vi "Image_Processing_Edge_Detection.vi"() -> ()   [LabVIEW 2015]
uses:
  <vilib>/picture/picture.llb/imagedata.ctl
  <vilib>/Analysis/2dsp.llb/2D Convolution (DBL).vi
  <vilib>/picture/picture.llb/Draw 8-Bit Pixmap.vi
  <vilib>/Analysis/NI_AALPro.lvlib
panel:
  out "new picture 2":picture
  out "new picture":picture
  out "image data":T1
  in  "Input Image":path
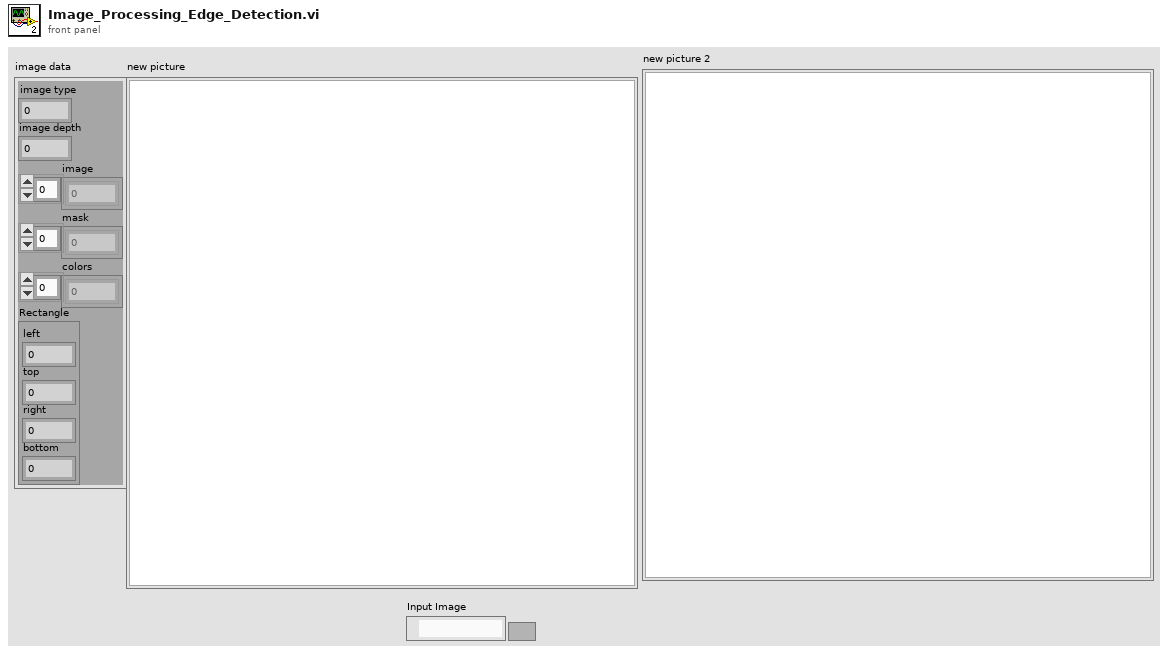
[diagram p1: front panel]
types:
  T1 = typedef "imagedata.ctl" = cluster{"image type":i32, "image depth":i32, "image":u8[], "mask":u8[], "colors":u32[], "Rectangle":cluster{"left":i16, "top":i16, "right":i16, "bottom":i16}}
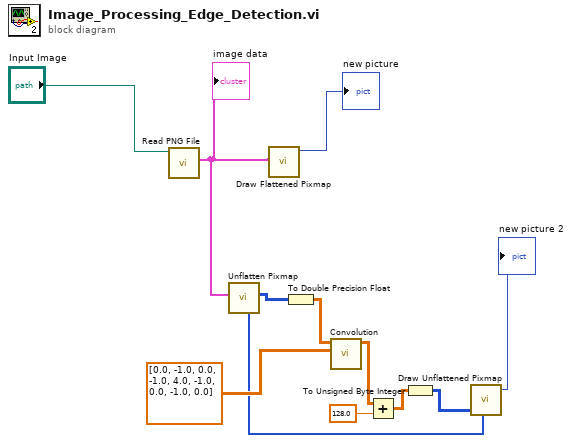
[diagram p0: block diagram]
diagram:
  n1 = call <vilib>:"Read PNG File.vi"("path to PNG file"="Input Image") -> ("image data"=w10:T1)  [unwired: 8 in, 2 out]
  "image data" <- w10
  n2 = call <vilib>:"Unflatten Pixmap.vi"("image data"=w10) -> ("8-bit pixmap"=w1:u8[][], "colors"=w2:u32[])  [unwired: 4 in, 5 out]
  n3 = call <vilib>:"Draw Flattened Pixmap.vi"("image data"=w10) -> ("new picture"=→"new picture":picture)  [unwired: 8 in]
  n4 = To Double Precision Float(number=w1) -> (double precision float=w9:dbl[][])
  n5 = call-poly <vilib>:"Convolution.vi"("Y"=dbl[][] [[0.0, -1.0, 0.0], [-1.0, 4.0, -1.0], [0.0, -1.0, 0.0]], "X"=w9) -> ("X * Y"=w5:dbl[][])  [unwired: 8 in, 1 out]
  n6 = Add(x=w5, y=128.0) -> (x+y=w7:dbl[][])
  n7 = To Unsigned Byte Integer(number=w7) -> (unsigned 8bit integer=w4:u8[][])
  n8 = call-poly <vilib>:"Draw Unflattened Pixmap.vi"("data"=w4, "color table"=w2) -> ("new picture"=→"new picture 2":picture)  [unwired: 7 in]
